vi "Append Chapter bookmark.vi"(0 "PDF Report":refnum<class "PDF Report Class.lvclass">, 1 "Chapter or section":T1, 2 "Title":string, 3 "Title indentation":T2, 5 "TriggerNewPage (Chapter)":bool=TRUE, 11 "error in (no error)":errorcluster, 12 "Font":T6={"Name"="", "Size"=-1.0, "Color"=0, "Style"={"Bold"=TRUE, "Italic"=FALSE, "Underline"=FALSE, "Strikeout"=FALSE}, "Type"={"Type&direction"=enum."Select", "Embedded"=FALSE, "Encoding"=""}}, 14 "Title properties":T3={" Aligment"=enum."LEFT", "Line spacing"=enum."Select"}) -> (4 "PDF Report duplicate":refnum<class "PDF Report Class.lvclass">, 15 "error out":errorcluster)   [LabVIEW 2020, in "Exaprom PDF.lvlib"]
doc: "<B>Only ASCII or UTF-16 (no-bidi).</B>\n\nAppends text with a <B>line feed</B>, at the end, to the PDF report. This text can be <B>aligned</B> (CENTER, JUSTIFY, LEFT, RIGHT) and <B>indented</B>. \n\nIf <B>Font</B> and <B>Pararaph properties</B> are not specified then the <B>Default font</B> and <B>Default paragraph</B> will be use.\n\nThe data type you wire to the <B>Text</B> input determines the polymorphic instance to use.\n\n<B>FRANÇAIS</B>\nAjoute au rapport PDF du texte sous la forme d'un paragraphe terminé avec un \"<B>Line Feed</B>\". Ce texte peut être <B>aligné</B> (CENTER, JUSTIFY, LEFT, RIGHT) et avoir un <B>renfoncement</B> (gauche et droit) pour tout le paragraphe.\n\nSi la police de caractères <B>Font</B> et les propriétés <B>Pararaph properties</B> ne sont pas spécifiés alors la police par défaut <B>Default font</B> et <B>Default paragraph</B> seront utilisées.\n\nLe type de données que vous connectez au terminal <B>Text</B> détermine l'instance polymorphique utilisée.\n\nVersion 2.0\nDeveloped by Jean-Marc Simard\nCopyright © 2013, Exaprom Inc.\nAll rights reserved.\nLicense: BSD\n\nWith iTextSharp 4.1.6 (http://itextsharp.sourceforge.net)\nunder Mozilla Public License Version 1.1\n(http://www.mozilla.org/MPL/MPL-1.1.html)"
uses:
  <userlib>/labview-PDF-writer-master/Exaprom PDF.lvlib
  <userlib>/labview-PDF-writer-master/Controls/Font Controls/Font complete cluster.ctl
  <userlib>/labview-PDF-writer-master/Controls/Font Controls/Font size.ctl
  <userlib>/labview-PDF-writer-master/Controls/Font Controls/Font color.ctl
  <userlib>/labview-PDF-writer-master/Controls/Font Controls/Type and encoding.ctl
  <userlib>/labview-PDF-writer-master/Controls/Text Controls/Unicode/Type and run direction.ctl
  <userlib>/labview-PDF-writer-master/Controls/Initialization Controls/Defaut Paragraphe and Line Spacing.ctl
  <userlib>/labview-PDF-writer-master/Controls/Text Controls/Texte alignement.ctl
  <userlib>/labview-PDF-writer-master/Controls/Text Controls/Line spacing.ctl
  <userlib>/labview-PDF-writer-master/LV Class/PDF Report Class/PDF Report Class.lvclass
  <userlib>/labview-PDF-writer-master/Controls/Text Controls/Paragraph indentation.ctl
  <userlib>/labview-PDF-writer-master/Controls/Chapter Controls/Chapter.ctl
  <userlib>/labview-PDF-writer-master/Controls/Text Controls/Phrase or paragraph.ctl
  <userlib>/labview-PDF-writer-master/Controls/Text Controls/Unicode/Source rub direction.ctl
  C:/Program Files (x86)/National Instruments/LabVIEW 2020/user.lib/labview-PDF-writer-master/DLL/itextsharp.dll
  DLL/itextsharp.dll
  <userlib>/labview-PDF-writer-master/LV Class/Fonts Class/Font Class.lvclass
panel:
  # "标题"
  # "标题缩进"
  # "章或节"
  # "Left 左\nRight 右"
  # "触发新页"
  # "字体"
  # "标题属性联系"
  # "Aligment 对齐\nLine spacing 行距"
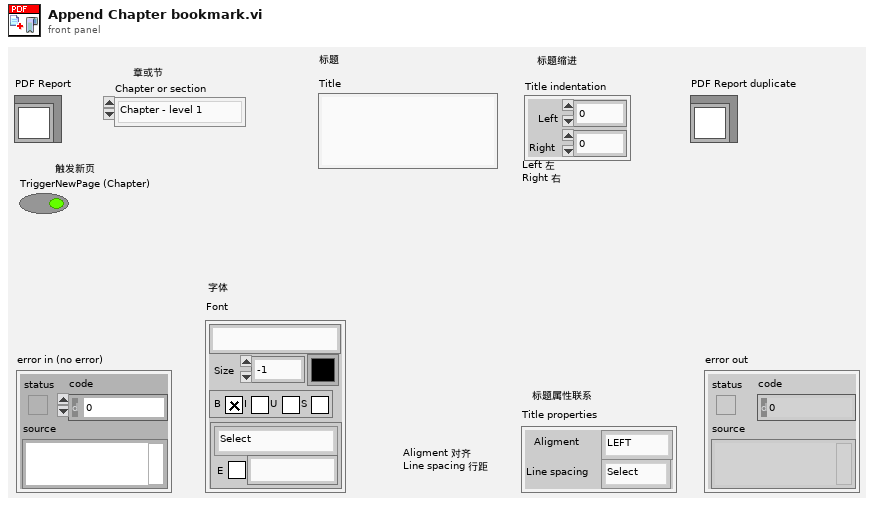
[diagram p1: front panel]
types:
  T1 = typedef "Exaprom PDF.lvlib/Chapter.ctl" = enum16{"Chapter - level 1", "Chapter - level 2", "Chapter - level 3", "Chapter - level 4"}
  T2 = typedef "Exaprom PDF.lvlib/Paragraph indentation.ctl" = cluster{"Left":sgl, "Right":sgl}
  T3 = typedef "Exaprom PDF.lvlib/Defaut Paragraphe and Line Spacing.ctl" = cluster{" Aligment":T4, "Line spacing":T5}
  T4 = typedef "Exaprom PDF.lvlib/Texte alignement.ctl" = enum16{"Select", "CENTER", "JUSTIFY", "LEFT", "RIGHT"}
  T5 = typedef "Exaprom PDF.lvlib/Line spacing.ctl" = enum16{"Select", "1.0", "1.5", "2.0"}
  T6 = typedef "Exaprom PDF.lvlib/Font complete cluster.ctl" = cluster{"Name":string, "Size":T7, "Color":T8, "Style":cluster{"Bold":bool, "Italic":bool, "Underline":bool, "Strikeout":bool}, "Type":T9}
  T7 = typedef "Exaprom PDF.lvlib/Font size.ctl" = sgl
  T8 = typedef "Exaprom PDF.lvlib/Font color.ctl" = u32
  T9 = typedef "Exaprom PDF.lvlib/Type and encoding.ctl" = cluster{"Type&direction":T10, "Embedded":bool, "Encoding":string}
  T10 = typedef "Exaprom PDF.lvlib/Type and run direction.ctl" = enum16{"Select", "ASCII", "UTF-16", "UTF-16 (default)", "UTF-16 (LTR)", "UTF-16 (RTL)"}
  T11 = typedef "Exaprom PDF.lvlib/Source rub direction.ctl" = enum16{"Chapter", "Paragraph", "Phrase", "pdfpcell"}
  T12 = typedef "Exaprom PDF.lvlib/Phrase or paragraph.ctl" = enum16{"Add to Phrase", "Add to Paragraph", "Create Phrase", "Create Paragraph"}
  T13 = typedef "Exaprom PDF.lvlib/Unit.ctl" = enum16{"inch", "mm"}
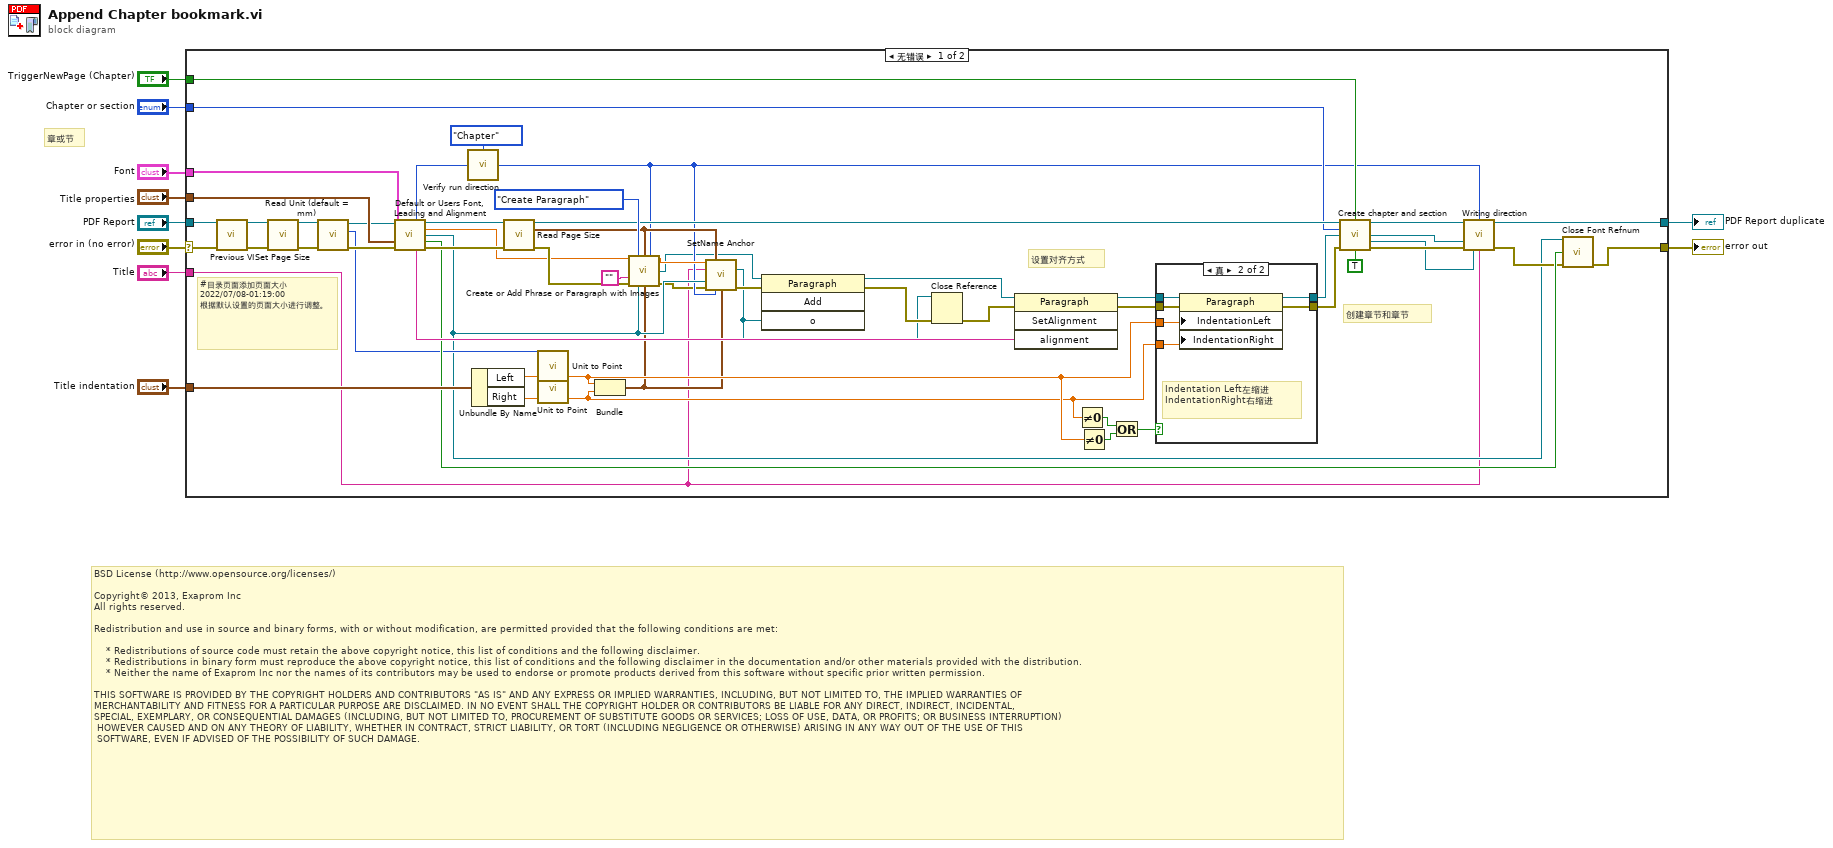
[diagram p0: block diagram]
diagram:
  # "章或节"
  # "BSD License (http://www.opensource.org/licenses/)\n\nCopyright© 2013, Exaprom Inc\nAll rights reserved.\n\nRedistribution and use in source and binary forms, with or without modification, are permitted provided that the following conditions are met:\n\n    * Redistributions of source code must retain the above copyright notice, this list of conditions and the following disclaimer.\n    * Redistributions in binary form must reproduce the above copyright notice, this list of conditions and the following disclaimer in the documentation and/or other materials provided with the distribution.\n    * Neither the name of Exaprom Inc nor the names of its contributors may be used to endorse or promote products derived from this software without specific prior written permission.\n\nTHIS SOFTWARE IS PROVIDED BY THE COPYRIGHT HOLDERS AND CONTRIBUTORS \"AS IS\" AND ANY EXPRESS OR IMPLIED WARRANTIES, INCLUDING, BUT NOT LIMITED TO, THE IMPLIED WARRANTIES OF \nMERCHANTABILITY AND FITNESS FOR A PARTICULAR PURPOSE ARE DISCLAIMED. IN NO EVENT SHALL THE COPYRIGHT HOLDER OR CONTRIBUTORS BE LIABLE FOR ANY DIRECT, INDIRECT, INCIDENTAL,\nSPECIAL, EXEMPLARY, OR CONSEQUENTIAL DAMAGES (INCLUDING, BUT NOT LIMITED TO, PROCUREMENT OF SUBSTITUTE GOODS OR SERVICES; LOSS OF USE, DATA, OR PROFITS; OR BUSINESS INTERRUPTION)\n HOWEVER CAUSED AND ON ANY THEORY OF LIABILITY, WHETHER IN CONTRACT, STRICT LIABILITY, OR TORT (INCLUDING NEGLIGENCE OR OTHERWISE) ARISING IN ANY WAY OUT OF THE USE OF THIS\n SOFTWARE, EVEN IF ADVISED OF THE POSSIBILITY OF SUCH DAMAGE."
  n1 = case shown="无错误" "error in (no error)" {
    selector: "error in (no error)" -> [w46 w76]
    tunnel: "Font" -> [w32 _]
    tunnel: "Title" -> [w22 _]
    tunnel: [w54 w76] -> w9
    tunnel: "PDF Report" -> [w58 w75]
    tunnel: "Title properties" -> [w57 _]
    tunnel: [w44 w75] -> w5
    tunnel: "Title indentation" -> [w64 _]
    tunnel: "TriggerNewPage (Chapter)" -> [w35 _]
    tunnel: "Chapter or section" -> [w34 _]
    frame No Error {
      # "创建章节和章节"
      # "设置对齐方式"
      # "#目录页面添加页面大小\n2022/07/08-01:19:00\n根据默认设置的页面大小进行调整。"
      n2 = call <userlib>:"Previous VI.vi"("PDF Report IN"=w58, "error in (no error)"=w46) -> ("PDF Report OUT"=w15:refnum<class "PDF Report Class.lvclass">, "error out"=w13:errorcluster)  [unwired: 12 out]
      n3 = call <userlib>:"Set Page Size.vi"("PDF Report IN"=w15, "error in (no error)"=w13) -> ("PDF Report OUT"=w14:refnum<class "PDF Report Class.lvclass">, "error OUT"=w12:errorcluster)  [unwired: 12 in]
      n4 = call-dynamic "Read Unit (default = mm).vi"("error in (no error)"=w12, "PDF Report Class in"=w14) -> ("error out"=w52:errorcluster, "Unit (default = mm)"=w50:T13, "PDF Report Class out"=w51:refnum<class "PDF Report Class.lvclass">)  [unwired: 7 in]
      n5 = call <userlib>:"Default or Users Font, Leading and Alignment.vi"("PDF Report"=w51, "Font"=w32, "Paragraphe cluster"=w57, "error in (no error)"=w52) -> ("Type and run direction"=w31:T10, "PDF Report duplicate"=w55:refnum<class "PDF Report Class.lvclass">, "Leading"=w27:T7, "Font Ref"=w26:refnum<k24>, "Close Font Ref"=w53:bool, "Aligment"=w66:string, "error out"=w56:errorcluster)  [unwired: 5 out]
      n6 = call <userlib>:"Verify run direction.vi"("Source"=Source_rub_direction."Chapter", "Type&direction IN"=w31) -> ("Type&direction OUT"=w25:T10)  [unwired: 2 in]
      n7 = Unbundle By Name(w64) -> ("Left"=w60:sgl, "Right"=w59:sgl)
      n8 = call <userlib>:"Read Page Size.vi"("PDF Report"=w55, "error in (no error)"=w56) -> ("PDF Report duplicate"=w43:refnum<class "PDF Report Class.lvclass">, "Text zone (points)"=w28:cluster{"widht":sgl, "height":sgl}, "error out"=w41:errorcluster)  [unwired: 11 out]
      n9 = call <userlib>:"Unit to Point.vi"("X unit"=w60, "Unit (default = mm)"=w50) -> ("X point"=w48:sgl)  [unwired: 7 out]
      n10 = call <userlib>:"Unit to Point.vi"("X unit"=w59, "Unit (default = mm)"=w50) -> ("X point"=w47:sgl)  [unwired: 7 out]
      n11 = Bundle("X point"=w48, "X point"=w47) -> (w24:cluster{" X point":sgl, " X point":sgl})  [unwired: 1 out]
      n12 = call <userlib>:"Create or Add Phrase or Paragraph with Images.vi"("Leading"=w27, "Phrase or paragraph"=Phrase_or_paragraph."Create Paragraph", "Text zone (points)"=w28, "Character type"=w25, "Text"="", "error in (no error)"=w41, "Font refnum"=w26, "Paragraph indentation (points)"=w24) -> ("Paragraph refnum OUT"=w17:refnum<k24>, "error out"=w23:errorcluster)  [unwired: 3 in, 3 out]
      n13 = call <userlib>:"SetName Anchor.vi"("Leading"=w27, "Text zone (points)"=w28, "Text"=w22, "Font refnum"=w26, "error in (no error)"=w23, "Type and run direction"=w25, "Paragraph indentation (points)"=w24) -> ("Anchor"=w11:refnum<k24>, "error out"=w21:errorcluster)  [unwired: 6 in, 1 out]
      n14 = invoke class="Paragraph" method="Add"(reference=w17, error in=w21, "o"=w11) -> (reference out=w19:refnum<k24>, error out=w20:errorcluster)  [unwired: 1 in, 2 out]
      n15 = Close Reference(reference=w11, error in (no error)=w20) -> (error out=w18:errorcluster)
      n16 = invoke class="Paragraph" method="SetAlignment"(reference=w19, error in=w18, "alignment"=w66) -> (reference out=w42:refnum<k24>, error out=w65:errorcluster)  [unwired: 1 in, 2 out]
      n17 = Not Equal To 0?(x=w47) -> (x != 0?=w62:bool)
      n18 = Not Equal To 0?(x=w48) -> (x != 0?=w61:bool)
      n19 = Or(x=w62, y=w61) -> (x .or. y?=w63:bool)
      n20 = case shown="真" w63 {
        tunnel: w42 -> [w68 w74]
        tunnel: w65 -> [w67 w73]
        tunnel: [w67 w72] -> w38
        tunnel: [w68 w71] -> w37
        tunnel: w48 -> [_ w70]
        tunnel: w47 -> [_ w69]
        frame False {
        }
        frame True {
          # "Indentation Left左缩进\nIndentationRight右缩进"
          n21 = property class="Paragraph"(reference=w74, error in=w73, "IndentationLeft"=w70, "IndentationRight"=w69) -> (reference out=w71:refnum<k24>, error out=w72:errorcluster)
        }
      }
      n22 = call <userlib>:"Create chapter and section.vi"("PDF Report IN"=w43, "TriggerNewPage"=w35, "Chapter or section IN"=w34, "Paragragh"=w37, "error in (no error)"=w38, "BookmarkOpen"=TRUE) -> ("PDF Report OUT"=w40:refnum<class "PDF Report Class.lvclass">, "Chapter"=w33:refnum<k24>, "Section"=w36:refnum<k24>, "error out"=w39:errorcluster)  [unwired: 6 in]
      n23 = call <userlib>:"Writing direction.vi"("PDF Report IN"=w40, "Text type"=w25, "ChapterAutoNumber"=w33, "error in (no error)"=w39, "Section"=w36, "Title"=w22) -> ("PDF Report OUT"=w44:refnum<class "PDF Report Class.lvclass">, "error out"=w45:errorcluster)  [unwired: 8 in]
      n24 = call <userlib>:"Close Font Refnum.vi"("Font Refnum"=w26, "Close ?"=w53, "error in (no error)"=w45) -> ("error out"=w54:errorcluster)  [unwired: 12 in]
    }
    frame Error {
    }
  }
  "error out" <- w9
  "PDF Report duplicate" <- w5
